vi "Send Notification Msg.vi"(8 "error in (no error)":errorcluster, 9 "Publication Time (Use Current Time)":timestamp, 10 "Value":variant, 11 "Notification Msg":refnum<class "Notification Msg.lvclass">) -> (0 "error out":errorcluster)   [LabVIEW 2020, in "ActorMessageTransport.lvlib" / "Notification Msg.lvclass"]
doc: "Sends Notification Msg back to originator.\n\n*** DO NOT OVERRIDE THIS METHOD ***\nDynamic Dispatch added to this method for backwards compatibility in MVA Framework. DD will be removed in a future release."
uses:
  Notification Msg.lvclass
  Notification Msg.lvclass/Notification Msg.ctl
  composed-af-messages/Source/RoundTripMessage/RoundTripMessage.lvclass/RoundTripMessage.ctl
  <vilib>/ActorFramework/Message Enqueuer/Message Enqueuer.lvclass/Message Enqueuer.ctl
  <vilib>/ActorFramework/Message Enqueuer/Enqueue.vi
  composed-af-messages/Source/RoundTripMessage/RoundTripMessage.lvclass
  C:/Program Files/National Instruments/LabVIEW 2020/vi.lib/ActorFramework/Message/Message.lvclass
  <vilib>/ActorFramework/Message Priority Queue/Priority Enqueue.vi
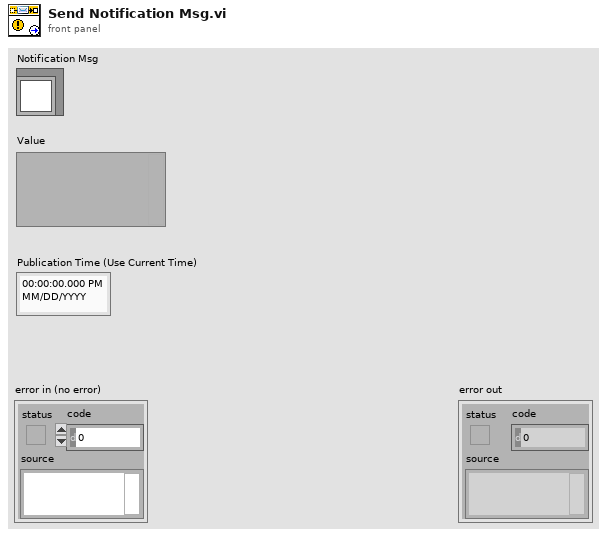
[diagram p1: front panel]
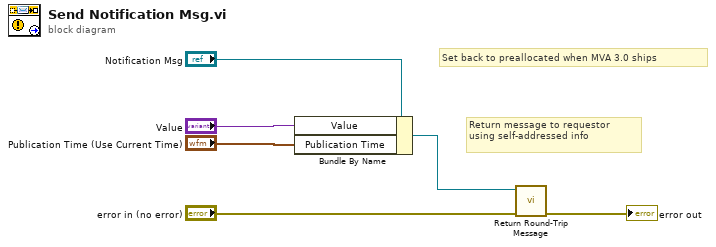
[diagram p0: block diagram]
diagram:
  # "Set back to preallocated when MVA 3.0 ships"
  # "Return message to requestor\nusing self-addressed info"
  n1 = Bundle By Name(cluster="Notification Msg", "Value"="Value", "Publication Time"="Publication Time (Use Current Time)") -> (w2:refnum<class "Notification Msg.lvclass">)
  n2 = call "Return Round-Trip Message.vi"("error in (no error)"="error in (no error)", "RoundTripMessage In"=w2) -> ("error out"=→"error out":errorcluster)  [unwired: 9 in]
